vi "getCurrentPosition.vi"(0 "reference (in)":refnum<class "_MultiAxisController.lvclass">, 2 "axis (in)":T1, 5 "error in (no error)":errorcluster) -> (14 "reference (out)":refnum<class "_MultiAxisController.lvclass">, 16 "current_position (units)":i32, 19 "error out":errorcluster)   [LabVIEW 2020, in "classes.lvlib" / "_MultiAxisController.lvclass"]
doc: "Produced By:\n\n<B>Kod Integrations, LLC</B>\n4835 Marianne Drive\nMount Airy, MD 21771\nhttp://www.kodintegrations.com\nemail: info@kodintegrations.com\nphone: (240) 687-1288"
uses:
  _MultiAxisController.lvclass
  C:/GEECS/Developers Version/source/Device Drivers/Newmark-NSC-A/Arcus Driver 3.0.0/ArcusUsbComm/classes/Controller/_Controller.lvclass
  common/controls/axis.ctl
  Controller/_Controller.lvclass
  libraries/common.lvlib
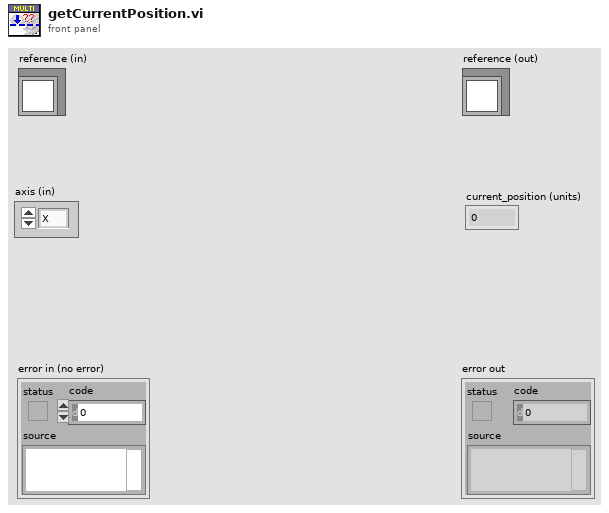
[diagram p1: front panel]
types:
  T1 = typedef "common.lvlib/axis.ctl" = enum16{"X", "Y", "Z", "U"}
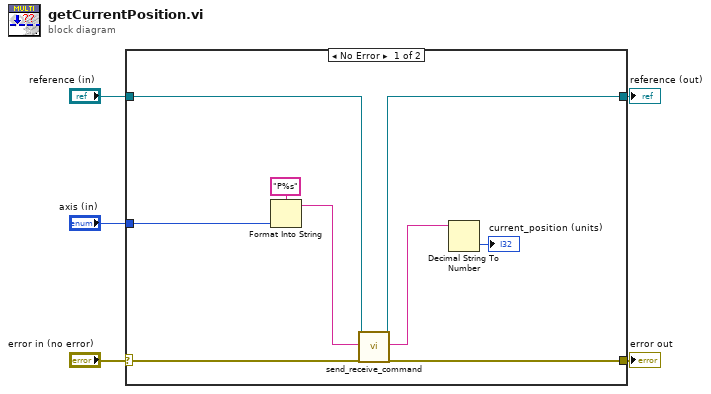
[diagram p0: block diagram]
diagram:
  n1 = case shown="No Error" "error in (no error)" {
    selector: "error in (no error)" -> [w12 w16]
    tunnel: [w11 w16] -> w4
    tunnel: [w9 w15] -> w2
    tunnel: "reference (in)" -> [w10 w15]
    tunnel: "axis (in)" -> [w7 _]
    frame No Error {
      n2 = Format Into String(format string="P%s" ("ASCII Command (in)"), w7) -> (resulting string=w6:string)  [unwired: 2 in, 1 out]
      n3 = call "send_receive_command.vi"("reference (in)"=w10, "ASCII Command (in)"=w6, "error in (no error)"=w12) -> ("reference (out)"=w9:refnum<class "_MultiAxisController.lvclass">, "response (out)"=w13:string, "error out"=w11:errorcluster)  [unwired: 12 in, 2 out]
      n4 = Decimal String To Number(string=w13) -> (number=→"current_position (units)":i32)  [unwired: 2 in, 1 out]
    }
    frame Error {
    }
  }
  "error out" <- w4
  "reference (out)" <- w2
